vi "FipsAdjacent.vi"() -> (11 "Fips":i32[](array[numeric]))   [LabVIEW 2017] (continued)
Perce County, ID\"\t16069\n\"Idaho County, ID\"\t16049\t\"Valley County, ID\"\t16085\n\"Idaho County, ID\"\t16049\t\"Missoula County, MT\"\t30063\n\"Idaho County, ID\"\t16049\t\"Ravalli County, MT\"\t30081\n\"Idaho County, ID\"\t16049\t\"Wallowa County, OR\"\t41063\n\"Jefferson County, ID\"\t16051\t\"Bingham County, ID\"\t16011\n\"Jefferson County, ID\"\t16051\t\"Bonneville County, ID\"\t16019\n\"Jefferson County, ID\"\t16051\t\"Butte County, ID\"\t16023\n\"Jefferson County, ID\"\t16051\t\"Clark County, ID\"\t16033\n\"Jefferson County, ID\"\t16051\t\"Fremont County, ID\"\t16043\n\"Jefferson County, ID\"\t16051\t\"Jefferson County, ID\"\t16051\n\"Jefferson County, ID\"\t16051\t\"Madison County, ID\"\t16065\n\"Jerome County, ID\"\t16053\t\"Cassia County, ID\"\t16031\n\"Jerome County, ID\"\t16053\t\"Gooding County, ID\"\t16047\n\"Jerome County, ID\"\t16053\t\"Jerome County, ID\"\t16053\n\"Jerome County, ID\"\t16053\t\"Lincoln County, ID\"\t16063\n\"Jerome County, ID\"\t16053\t\"Minidoka County, ID\"\t16067\n\"Jerome County, ID\"\t16053\t\"Twin Falls County, ID\"\t16083\n\"Kootenai County, ID\"\t16055\t\"Benewah County, ID\"\t16009\n\"Kootenai County, ID\"\t16055\t\"Bonner County, ID\"\t16017\n\"Kootenai County, ID\"\t16055\t\"Kootenai County, ID\"\t16055\n\"Kootenai County, ID\"\t16055\t\"Shoshone County, ID\"\t16079\n\"Kootenai County, ID\"\t16055\t\"Spokane County, WA\"\t53063\n\"Latah County, ID\"\t16057\t\"Benewah County, ID\"\t16009\n\"Latah County, ID\"\t16057\t\"Clearwater County, ID\"\t16035\n\"Latah County, ID\"\t16057\t\"Latah County, ID\"\t16057\n\"Latah County, ID\"\t16057\t\"Nez Perce County, ID\"\t16069\n\"Latah County, ID\"\t16057\t\"Shoshone County, ID\"\t16079\n\"Latah County, ID\"\t16057\t\"Whitman County, WA\"\t53075\n\"Lemhi County, ID\"\t16059\t\"Butte County, ID\"\t16023\n\"Lemhi County, ID\"\t16059\t\"Clark County, ID\"\t16033\n\"Lemhi County, ID\"\t16059\t\"Custer County, ID\"\t16037\n\"Lemhi County, ID\"\t16059\t\"Idaho County, ID\"\t16049\n\"Lemhi County, ID\"\t16059\t\"Lemhi County, ID\"\t16059\n\"Lemhi County, ID\"\t16059\t\"Valley County, ID\"\t16085\n\"Lemhi County, ID\"\t16059\t\"Beaverhead County, MT\"\t30001\n\"Lemhi County, ID\"\t16059\t\"Ravalli County, MT\"\t30081\n\"Lewis County, ID\"\t16061\t\"Clearwater County, ID\"\t16035\n\"Lewis County, ID\"\t16061\t\"Idaho County, ID\"\t16049\n\"Lewis County, ID\"\t16061\t\"Lewis County, ID\"\t16061\n\"Lewis County, ID\"\t16061\t\"Nez Perce County, ID\"\t16069\n\"Lincoln County, ID\"\t16063\t\"Blaine County, ID\"\t16013\n\"Lincoln County, ID\"\t16063\t\"Camas County, ID\"\t16025\n\"Lincoln County, ID\"\t16063\t\"Gooding County, ID\"\t16047\n\"Lincoln County, ID\"\t16063\t\"Jerome County, ID\"\t16053\n\"Lincoln County, ID\"\t16063\t\"Lincoln County, ID\"\t16063\n\"Lincoln County, ID\"\t16063\t\"Minidoka County, ID\"\t16067\n\"Madison County, ID\"\t16065\t\"Bonneville County, ID\"\t16019\n\"Madison County, ID\"\t16065\t\"Fremont County, ID\"\t16043\n\"Madison County, ID\"\t16065\t\"Jefferson County, ID\"\t16051\n\"Madison County, ID\"\t16065\t\"Madison County, ID\"\t16065\n\"Madison County, ID\"\t16065\t\"Teton County, ID\"\t16081\n\"Minidoka County, ID\"\t16067\t\"Blaine County, ID\"\t16013\n\"Minidoka County, ID\"\t16067\t\"Cassia County, ID\"\t16031\n\"Minidoka County, ID\"\t16067\t\"Jerome County, ID\"\t16053\n\"Minidoka County, ID\"\t16067\t\"Lincoln County, ID\"\t16063\n\"Minidoka County, ID\"\t16067\t\"Minidoka County, ID\"\t16067\n\"Nez Perce County, ID\"\t16069\t\"Clearwater County, ID\"\t16035\n\"Nez Perce County, ID\"\t16069\t\"Idaho County, ID\"\t16049\n\"Nez Perce County, ID\"\t16069\t\"Latah County, ID\"\t16057\n\"Nez Perce County, ID\"\t16069\t\"Lewis County, ID\"\t16061\n\"Nez Perce County, ID\"\t16069\t\"Nez Perce County, ID\"\t16069\n\"Nez Perce County, ID\"\t16069\t\"Wallowa County, OR\"\t41063\n\"Nez Perce County, ID\"\t16069\t\"Asotin County, WA\"\t53003\n\"Nez Perce County, ID\"\t16069\t\"Whitman County, WA\"\t53075\n\"Oneida County, ID\"\t16071\t\"Bannock County, ID\"\t16005\n\"Oneida County, ID\"\t16071\t\"Cassia County, ID\"\t16031\n\"Oneida County, ID\"\t16071\t\"Franklin County, ID\"\t16041\n\"Oneida County, ID\"\t16071\t\"Oneida County, ID\"\t16071\n\"Oneida County, ID\"\t16071\t\"Power County, ID\"\t16077\n\"Oneida County, ID\"\t16071\t\"Box Elder County, UT\"\t49003\n\"Oneida County, ID\"\t16071\t\"Cache County, UT\"\t49005\n\"Owyhee County, ID\"\t16073\t\"Ada County, ID\"\t16001\n\"Owyhee County, ID\"\t16073\t\"Canyon County, ID\"\t16027\n\"Owyhee County, ID\"\t16073\t\"Elmore County, ID\"\t16039\n\"Owyhee County, ID\"\t16073\t\"Owyhee County, ID\"\t16073\n\"Owyhee County, ID\"\t16073\t\"Twin Falls County, ID\"\t16083\n\"Owyhee County, ID\"\t16073\t\"Elko County, NV\"\t32007\n\"Owyhee County, ID\"\t16073\t\"Humboldt County, NV\"\t32013\n\"Owyhee County, ID\"\t16073\t\"Malheur County, OR\"\t41045\n\"Payette County, ID\"\t16075\t\"Canyon County, ID\"\t16027\n\"Payette County, ID\"\t16075\t\"Gem County, ID\"\t16045\n\"Payette County, ID\"\t16075\t\"Payette County, ID\"\t16075\n\"Payette County, ID\"\t16075\t\"Washington County, ID\"\t16087\n\"Payette County, ID\"\t16075\t\"Malheur County, OR\"\t41045\n\"Power County, ID\"\t16077\t\"Bannock County, ID\"\t16005\n\"Power County, ID\"\t16077\t\"Bingham County, ID\"\t16011\n\"Power County, ID\"\t16077\t\"Blaine County, ID\"\t16013\n\"Power County, ID\"\t16077\t\"Cassia County, ID\"\t16031\n\"Power County, ID\"\t16077\t\"Oneida County, ID\"\t16071\n\"Power County, ID\"\t16077\t\"Power County, ID\"\t16077\n\"Shoshone County, ID\"\t16079\t\"Benewah County, ID\"\t16009\n\"Shoshone County, ID\"\t16079\t\"Bonner County, ID\"\t16017\n\"Shoshone County, ID\"\t16079\t\"Clearwater County, ID\"\t16035\n\"Shoshone County, ID\"\t16079\t\"Kootenai County, ID\"\t16055\n\"Shoshone County, ID\"\t16079\t\"Latah County, ID\"\t16057\n\"Shoshone County, ID\"\t16079\t\"Shoshone County, ID\"\t16079\n\"Shoshone County, ID\"\t16079\t\"Mineral County, MT\"\t30061\n\"Shoshone County, ID\"\t16079\t\"Sanders County, MT\"\t30089\n\"Teton County, ID\"\t16081\t\"Bonneville County, ID\"\t16019\n\"Teton County, ID\"\t16081\t\"Fremont County, ID\"\t16043\n\"Teton County, ID\"\t16081\t\"Madison County, ID\"\t16065\n\"Teton County, ID\"\t16081\t\"Teton County, ID\"\t16081\n\"Teton County, ID\"\t16081\t\"Teton County, WY\"\t56039\n\"Twin Falls County, ID\"\t16083\t\"Cassia County, ID\"\t16031\n\"Twin Falls County, ID\"\t16083\t\"Elmore County, ID\"\t16039\n\"Twin Falls County, ID\"\t16083\t\"Gooding County, ID\"\t16047\n\"Twin Falls County, ID\"\t16083\t\"Jerome County, ID\"\t16053\n\"Twin Falls County, ID\"\t16083\t\"Owyhee County, ID\"\t16073\n\"Twin Falls County, ID\"\t16083\t\"Twin Falls County, ID\"\t16083\n\"Twin Falls County, ID\"\t16083\t\"Elko County, NV\"\t32007\n\"Valley County, ID\"\t16085\t\"Adams County, ID\"\t16003\n\"Valley County, ID\"\t16085\t\"Boise County, ID\"\t16015\n\"Valley County, ID\"\t16085\t\"Custer County, ID\"\t16037\n\"Valley County, ID\"\t16085\t\"Gem County, ID\"\t16045\n\"Valley County, ID\"\t16085\t\"Idaho County, ID\"\t16049\n\"Valley County, ID\"\t16085\t\"Lemhi County, ID\"\t16059\n\"Valley County, ID\"\t16085\t\"Valley County, ID\"\t16085\n\"Washington County, ID\"\t16087\t\"Adams County, ID\"\t16003\n\"Washington County, ID\"\t16087\t\"Gem County, ID\"\t16045\n\"Washington County, ID\"\t16087\t\"Payette County, ID\"\t16075\n\"Washington County, ID\"\t16087\t\"Washington County, ID\"\t16087\n\"Washington County, ID\"\t16087\t\"Baker County, OR\"\t41001\n\"Washington County, ID\"\t16087\t\"Malheur County, OR\"\t41045\n\"Adams County, IL\"\t17001\t\"Adams County, IL\"\t17001\n\"Adams County, IL\"\t17001\t\"Brown County, IL\"\t17009\n\"Adams County, IL\"\t17001\t\"Hancock County, IL\"\t17067\n\"Adams County, IL\"\t17001\t\"Pike County, IL\"\t17149\n\"Adams County, IL\"\t17001\t\"Schuyler County, IL\"\t17169\n\"Adams County, IL\"\t17001\t\"Lewis County, MO\"\t29111\n\"Adams County, IL\"\t17001\t\"Marion County, MO\"\t29127\n\"Alexander County, IL\"\t17003\t\"Alexander County, IL\"\t17003\n\"Alexander County, IL\"\t17003\t\"Pulaski County, IL\"\t17153\n\"Alexander County, IL\"\t17003\t\"Union County, IL\"\t17181\n\"Alexander County, IL\"\t17003\t\"Ballard County, KY\"\t21007\n\"Alexander County, IL\"\t17003\t\"Cape Girardeau County, MO\"\t29031\n\"Alexander County, IL\"\t17003\t\"Mississippi County, MO\"\t29133\n\"Alexander County, IL\"\t17003\t\"Scott County, MO\"\t29201\n\"Bond County, IL\"\t17005\t\"Bond County, IL\"\t17005\n\"Bond County, IL\"\t17005\t\"Clinton County, IL\"\t17027\n\"Bond County, IL\"\t17005\t\"Fayette County, IL\"\t17051\n\"Bond County, IL\"\t17005\t\"Madison County, IL\"\t17119\n\"Bond County, IL\"\t17005\t\"Montgomery County, IL\"\t17135\n\"Boone County, IL\"\t17007\t\"Boone County, IL\"\t17007\n\"Boone County, IL\"\t17007\t\"DeKalb County, IL\"\t17037\n\"Boone County, IL\"\t17007\t\"McHenry County, IL\"\t17111\n\"Boone County, IL\"\t17007\t\"Ogle County, IL\"\t17141\n\"Boone County, IL\"\t17007\t\"Winnebago County, IL\"\t17201\n\"Boone County, IL\"\t17007\t\"Rock County, WI\"\t55105\n\"Boone County, IL\"\t17007\t\"Walworth County, WI\"\t55127\n\"Brown County, IL\"\t17009\t\"Adams County, IL\"\t17001\n\"Brown County, IL\"\t17009\t\"Brown County, IL\"\t17009\n\"Brown County, IL\"\t17009\t\"Cass County, IL\"\t17017\n\"Brown County, IL\"\t17009\t\"Morgan County, IL\"\t17137\n\"Brown County, IL\"\t17009\t\"Pike County, IL\"\t17149\n\"Brown County, IL\"\t17009\t\"Schuyler County, IL\"\t17169\n\"Bureau County, IL\"\t17011\t\"Bureau County, IL\"\t17011\n\"Bureau County, IL\"\t17011\t\"Henry County, IL\"\t17073\n\"Bureau County, IL\"\t17011\t\"LaSalle County, IL\"\t17099\n\"Bureau County, IL\"\t17011\t\"Lee County, IL\"\t17103\n\"Bureau County, IL\"\t17011\t\"Marshall County, IL\"\t17123\n\"Bureau County, IL\"\t17011\t\"Putnam County, IL\"\t17155\n\"Bureau County, IL\"\t17011\t\"Stark County, IL\"\t17175\n\"Bureau County, IL\"\t17011\t\"Whiteside County, IL\"\t17195\n\"Calhoun County, IL\"\t17013\t\"Calhoun County, IL\"\t17013\n\"Calhoun County, IL\"\t17013\t\"Greene County, IL\"\t17061\n\"Calhoun County, IL\"\t17013\t\"Jersey County, IL\"\t17083\n\"Calhoun County, IL\"\t17013\t\"Pike County, IL\"\t17149\n\"Calhoun County, IL\"\t17013\t\"Lincoln County, MO\"\t29113\n\"Calhoun County, IL\"\t17013\t\"Pike County, MO\"\t29163\n\"Calhoun County, IL\"\t17013\t\"St. Charles County, MO\"\t29183\n\"Carroll County, IL\"\t17015\t\"Carroll County, IL\"\t17015\n\"Carroll County, IL\"\t17015\t\"Jo Daviess County, IL\"\t17085\n\"Carroll County, IL\"\t17015\t\"Ogle County, IL\"\t17141\n\"Carroll County, IL\"\t17015\t\"Stephenson County, IL\"\t17177\n\"Carroll County, IL\"\t17015\t\"Whiteside County, IL\"\t17195\n\"Carroll County, IL\"\t17015\t\"Clinton County, IA\"\t19045\n\"Carroll County, IL\"\t17015\t\"Jackson County, IA\"\t19097\n\"Cass County, IL\"\t17017\t\"Brown County, IL\"\t17009\n\"Cass County, IL\"\t17017\t\"Cass County, IL\"\t17017\n\"Cass County, IL\"\t17017\t\"Mason County, IL\"\t17125\n\"Cass County, IL\"\t17017\t\"Menard County, IL\"\t17129\n\"Cass County, IL\"\t17017\t\"Morgan County, IL\"\t17137\n\"Cass County, IL\"\t17017\t\"Sangamon County, IL\"\t17167\n\"Cass County, IL\"\t17017\t\"Schuyler County, IL\"\t17169\n\"Champaign County, IL\"\t17019\t\"Champaign County, IL\"\t17019\n\"Champaign County, IL\"\t17019\t\"Douglas County, IL\"\t17041\n\"Champaign County, IL\"\t17019\t\"Edgar County, IL\"\t17045\n\"Champaign County, IL\"\t17019\t\"Ford County, IL\"\t17053\n\"Champaign County, IL\"\t17019\t\"McLean County, IL\"\t17113\n\"Champaign County, IL\"\t17019\t\"Piatt County, IL\"\t17147\n\"Champaign County, IL\"\t17019\t\"Vermilion County, IL\"\t17183\n\"Christian County, IL\"\t17021\t\"Christian County, IL\"\t17021\n\"Christian County, IL\"\t17021\t\"Macon County, IL\"\t17115\n\"Christian County, IL\"\t17021\t\"Montgomery County, IL\"\t17135\n\"Christian County, IL\"\t17021\t\"Sangamon County, IL\"\t17167\n\"Christian County, IL\"\t17021\t\"Shelby County, IL\"\t17173\n\"Clark County, IL\"\t17023\t\"Clark County, IL\"\t17023\n\"Clark County, IL\"\t17023\t\"Coles County, IL\"\t17029\n\"Clark County, IL\"\t17023\t\"Crawford County, IL\"\t17033\n\"Clark County, IL\"\t17023\t\"Cumberland County, IL\"\t17035\n\"Clark County, IL\"\t17023\t\"Edgar County, IL\"\t17045\n\"Clark County, IL\"\t17023\t\"Jasper County, IL\"\t17079\n\"Clark County, IL\"\t17023\t\"Sullivan County, IN\"\t18153\n\"Clark County, IL\"\t17023\t\"Vigo County, IN\"\t18167\n\"Clay County, IL\"\t17025\t\"Clay County, IL\"\t17025\n\"Clay County, IL\"\t17025\t\"Effingham County, IL\"\t17049\n\"Clay County, IL\"\t17025\t\"Fayette County, IL\"\t17051\n\"Clay County, IL\"\t17025\t\"Jasper County, IL\"\t17079\n\"Clay County, IL\"\t17025\t\"Marion County, IL\"\t17121\n\"Clay County, IL\"\t17025\t\"Richland County, IL\"\t17159\n\"Clay County, IL\"\t17025\t\"Wayne County, IL\"\t17191\n\"Clinton County, IL\"\t17027\t\"Bond County, IL\"\t17005\n\"Clinton County, IL\"\t17027\t\"Clinton County, IL\"\t17027\n\"Clinton County, IL\"\t17027\t\"Fayette County, IL\"\t17051\n\"Clinton County, IL\"\t17027\t\"Madison County, IL\"\t17119\n\"Clinton County, IL\"\t17027\t\"Marion County, IL\"\t17121\n\"Clinton County, IL\"\t17027\t\"St. Clair County, IL\"\t17163\n\"Clinton County, IL\"\t17027\t\"Washington County, IL\"\t17189\n\"Coles County, IL\"\t17029\t\"Clark County, IL\"\t17023\n\"Coles County, IL\"\t17029\t\"Coles County, IL\"\t17029\n\"Coles County, IL\"\t17029\t\"Cumberland County, IL\"\t17035\n\"Coles County, IL\"\t17029\t\"Douglas County, IL\"\t17041\n\"Coles County, IL\"\t17029\t\"Edgar County, IL\"\t17045\n\"Coles County, IL\"\t17029\t\"Moultrie County, IL\"\t17139\n\"Coles County, IL\"\t17029\t\"Shelby County, IL\"\t17173\n\"Cook County, IL\"\t17031\t\"Cook County, IL\"\t17031\n\"Cook County, IL\"\t17031\t\"DuPage County, IL\"\t17043\n\"Cook County, IL\"\t17031\t\"Kane County, IL\"\t17089\n\"Cook County, IL\"\t17031\t\"Lake County, IL\"\t17097\n\"Cook County, IL\"\t17031\t\"McHenry County, IL\"\t17111\n\"Cook County, IL\"\t17031\t\"Will County, IL\"\t17197\n\"Cook County, IL\"\t17031\t\"Lake County, IN\"\t18089\n\"Cook County, IL\"\t17031\t\"Porter County, IN\"\t18127\n\"Cook County, IL\"\t17031\t\"Berrien County, MI\"\t26021\n\"Crawford County, IL\"\t17033\t\"Clark County, IL\"\t17023\n\"Crawford County, IL\"\t17033\t\"Crawford County, IL\"\t17033\n\"Crawford County, IL\"\t17033\t\"Jasper County, IL\"\t17079\n\"Crawford County, IL\"\t17033\t\"Lawrence County, IL\"\t17101\n\"Crawford County, IL\"\t17033\t\"Richland County, IL\"\t17159\n\"Crawford County, IL\"\t17033\t\"Knox County, IN\"\t18083\n\"Crawford County, IL\"\t17033\t\"Sullivan County, IN\"\t18153\n\"Cumberland County, IL\"\t17035\t\"Clark County, IL\"\t17023\n\"Cumberland County, IL\"\t17035\t\"Coles County, IL\"\t17029\n\"Cumberland County, IL\"\t17035\t\"Cumberland County, IL\"\t17035\n\"Cumberland County, IL\"\t17035\t\"Effingham County, IL\"\t17049\n\"Cumberland County, IL\"\t17035\t\"Jasper County, IL\"\t17079\n\"Cumberland County, IL\"\t17035\t\"Shelby County, IL\"\t17173\n\"DeKalb County, IL\"\t17037\t\"Boone County, IL\"\t17007\n\"DeKalb County, IL\"\t17037\t\"DeKalb County, IL\"\t17037\n\"DeKalb County, IL\"\t17037\t\"Kane County, IL\"\t17089\n\"DeKalb County, IL\"\t17037\t\"Kendall County, IL\"\t17093\n\"DeKalb County, IL\"\t17037\t\"LaSalle County, IL\"\t17099\n\"DeKalb County, IL\"\t17037\t\"Lee County, IL\"\t17103\n\"DeKalb County, IL\"\t17037\t\"McHenry County, IL\"\t17111\n\"DeKalb County, IL\"\t17037\t\"Ogle County, IL\"\t17141\n\"DeKalb County, IL\"\t17037\t\"Winnebago County, IL\"\t17201\n\"De Witt County, IL\"\t17039\t\"De Witt County, IL\"\t17039\n\"De Witt County, IL\"\t17039\t\"Logan County, IL\"\t17107\n\"De Witt County, IL\"\t17039\t\"McLean County, IL\"\t17113\n\"De Witt County, IL\"\t17039\t\"Macon County, IL\"\t17115\n\"De Witt County, IL\"\t17039\t\"Piatt County, IL\"\t17147\n\"Douglas County, IL\"\t17041\t\"Champaign County, IL\"\t17019\n\"Douglas County, IL\"\t17041\t\"Coles County, IL\"\t17029\n\"Douglas County, IL\"\t17041\t\"Douglas County, IL\"\t17041\n\"Douglas County, IL\"\t17041\t\"Edgar County, IL\"\t17045\n\"Douglas County, IL\"\t17041\t\"Moultrie County, IL\"\t17139\n\"Douglas County, IL\"\t17041\t\"Piatt County, IL\"\t17147\n\"Douglas County, IL\"\t17041\t\"Vermilion County, IL\"\t17183\n\"DuPage County, IL\"\t17043\t\"Cook County, IL\"\t17031\n\"DuPage County, IL\"\t17043\t\"DuPage County, IL\"\t17043\n\"DuPage County, IL\"\t17043\t\"Kane County, IL\"\t17089\n\"DuPage County, IL\"\t17043\t\"Kendall County, IL\"\t17093\n\"DuPage County, IL\"\t17043\t\"Will County, IL\"\t17197\n\"Edgar County, IL\"\t17045\t\"Champaign County, IL\"\t17019\n\"Edgar County, IL\"\t17045\t\"Clark County, IL\"\t17023\n\"Edgar County, IL\"\t17045\t\"Coles County, IL\"\t17029\n\"Edgar County, IL\"\t17045\t\"Douglas County, IL\"\t17041\n\"Edgar County, IL\"\t17045\t\"Edgar County, IL\"\t17045\n\"Edgar County, IL\"\t17045\t\"Vermilion County, IL\"\t17183\n\"Edgar County, IL\"\t17045\t\"Vermillion County, IN\"\t18165\n\"Edgar County, IL\"\t17045\t\"Vigo County, IN\"\t18167\n\"Edwards County, IL\"\t17047\t\"Edwards County, IL\"\t17047\n\"Edwards County, IL\"\t17047\t\"Richland County, IL\"\t17159\n\"Edwards County, IL\"\t17047\t\"Wabash County, IL\"\t17185\n\"Edwards County, IL\"\t17047\t\"Wayne County, IL\"\t17191\n\"Edwards County, IL\"\t17047\t\"White County, IL\"\t17193\n\"Effingham County, IL\"\t17049\t\"Clay County, IL\"\t17025\n\"Effingham County, IL\"\t17049\t\"Cumberland County, IL\"\t17035\n\"Effingham County, IL\"\t17049\t\"Effingham County, IL\"\t17049\n\"Effingham County, IL\"\t17049\t\"Fayette County, IL\"\t17051\n\"Effingham County, IL\"\t17049\t\"Jasper County, IL\"\t17079\n\"Effingham County, IL\"\t17049\t\"Shelby County, IL\"\t17173\n\"Fayette County, IL\"\t17051\t\"Bond County, IL\"\t17005\n\"Fayette County, IL\"\t17051\t\"Clay County, IL\"\t17025\n\"Fayette County, IL\"\t17051\t\"Clinton County, IL\"\t17027\n\"Fayette County, IL\"\t17051\t\"Effingham County, IL\"\t17049\n\"Fayette County, IL\"\t17051\t\"Fayette County, IL\"\t17051\n\"Fayette County, IL\"\t17051\t\"Marion County, IL\"\t17121\n\"Fayette County, IL\"\t17051\t\"Montgomery County, IL\"\t17135\n\"Fayette County, IL\"\t17051\t\"Shelby County, IL\"\t17173\n\"Ford County, IL\"\t17053\t\"Champaign County, IL\"\t17019\n\"Ford County, IL\"\t17053\t\"Ford County, IL\"\t17053\n\"Ford County, IL\"\t17053\t\"Iroquois County, IL\"\t17075\n\"Ford County, IL\"\t17053\t\"Kankakee County, IL\"\t17091\n\"Ford County, IL\"\t17053\t\"Livingston County, IL\"\t17105\n\"Ford County, IL\"\t17053\t\"McLean County, IL\"\t17113\n\"Ford County, IL\"\t17053\t\"Vermilion County, IL\"\t17183\n\"Franklin County, IL\"\t17055\t\"Franklin County, IL\"\t17055\n\"Franklin County, IL\"\t17055\t\"Hamilton County, IL\"\t17065\n\"Franklin County, IL\"\t17055\t\"Jackson County, IL\"\t17077\n\"Franklin County, IL\"\t17055\t\"Jefferson County, IL\"\t17081\n\"Franklin County, IL\"\t17055\t\"Perry County, IL\"\t17145\n\"Franklin County, IL\"\t17055\t\"Saline County, IL\"\t17165\n\"Franklin County, IL\"\t17055\t\"Williamson County, IL\"\t17199\n\"Fulton County, IL\"\t17057\t\"Fulton County, IL\"\t17057\n\"Fulton County, IL\"\t17057\t\"Knox County, IL\"\t17095\n\"Fulton County, IL\"\t17057\t\"McDonough County, IL\"\t17109\n\"Fulton County, IL\"\t17057\t\"Mason County, IL\"\t17125\n\"Fulton County, IL\"\t17057\t\"Peoria County, IL\"\t17143\n\"Fulton County, IL\"\t17057\t\"Schuyler County, IL\"\t17169\n\"Fulton County, IL\"\t17057\t\"Tazewell County, IL\"\t17179\n\"Fulton County, IL\"\t17057\t\"Warren County, IL\"\t17187\n\"Gallatin County, IL\"\t17059\t\"Gallatin County, IL\"\t17059\n\"Gallatin County, IL\"\t17059\t\"Hamilton County, IL\"\t17065\n\"Gallatin County, IL\"\t17059\t\"Hardin County, IL\"\t17069\n\"Gallatin County, IL\"\t17059\t\"Saline County, IL\"\t17165\n\"Gallatin County, IL\"\t17059\t\"White County, IL\"\t17193\n\"Gallatin County, IL\"\t17059\t\"Posey County, IN\"\t18129\n\"Gallatin County, IL\"\t17059\t\"Union County, KY\"\t21225\n\"Greene County, IL\"\t17061\t\"Calhoun County, IL\"\t17013\n\"Greene County, IL\"\t17061\t\"Greene County, IL\"\t17061\n\"Greene County, IL\"\t17061\t\"Jersey County, IL\"\t17083\n\"Greene County, IL\"\t17061\t\"Macoupin County, IL\"\t17117\n\"Greene County, IL\"\t17061\t\"Morgan County, IL\"\t17137\n\"Greene County, IL\"\t17061\t\"Pike County, IL\"\t17149\n\"Greene County, IL\"\t17061\t\"Scott County, IL\"\t17171\n\"Grundy County, IL\"\t17063\t\"Grundy County, IL\"\t17063\n\"Grundy County, IL\"\t17063\t\"Kankakee County, IL\"\t17091\n\"Grundy County, IL\"\t17063\t\"Kendall County, IL\"\t17093\n\"Grundy County, IL\"\t17063\t\"LaSalle County, IL\"\t17099\n\"Grundy County, IL\"\t17063\t\"Livingston County, IL\"\t17105\n\"Grundy County, IL\"\t17063\t\"Will County, IL\"\t17197\n\"Hamilton County, IL\"\t17065\t\"Franklin County, IL\"\t17055\n\"Hamilton County, IL\"\t17065\t\"Gallatin County, IL\"\t17059\n\"Hamilton County, IL\"\t17065\t\"Hamilton County, IL\"\t17065\n\"Hamilton County, IL\"\t17065\t\"Jefferson County, IL\"\t17081\n\"Hamilton County, IL\"\t17065\t\"Saline County, IL\"\t17165\n\"Hamilton County, IL\"\t17065\t\"Wayne County, IL\"\t17191\n\"Hamilton County, IL\"\t17065\t\"White County, IL\"\t17193\n\"Hancock County, IL\"\t17067\t\"Adams County, IL\"\t17001\n\"Hancock County, IL\"\t17067\t\"Hancock County, IL\"\t17067\n\"Hancock County, IL\"\t17067\t\"Henderson County, IL\"\t17071\n\"Hancock County, IL\"\t17067\t\"McDonough County, IL\"\t17109\n\"Hancock County, IL\"\t17067\t\"Schuyler County, IL\"\t17169\n\"Hancock County, IL\"\t17067\t\"Lee County, IA\"\t19111\n\"Hancock County, IL\"\t17067\t\"Clark County, MO\"\t29045\n\"Hancock County, IL\"\t17067\t\"Lewis County, MO\"\t29111\n\"Hardin County, IL\"\t17069\t\"Gallatin County, IL\"\t17059\n\"Hardin County, IL\"\t17069\t\"Hardin County, IL\"\t17069\n\"Hardin County, IL\"\t17069\t\"Pope County, IL\"\t17151\n\"Hardin County, IL\"\t17069\t\"Saline County, IL\"\t17165\n\"Hardin County, IL\"\t17069\t\"Crittenden County, KY\"\t21055\n\"Hardin County, IL\"\t17069\t\"Livingston County, KY\"\t21139\n\"Hardin County, IL\"\t17069\t\"Union County, KY\"\t21225\n\"Henderson County, IL\"\t17071\t\"Hancock County, IL\"\t17067\n\"Henderson County, IL\"\t17071\t\"Henderson County, IL\"\t17071\n\"Henderson County, IL\"\t17071\t\"McDonough County, IL\"\t17109\n\"Henderson County, IL\"\t17071\t\"Mercer County, IL\"\t17131\n\"Henderson County, IL\"\t17071\t\"Warren County, IL\"\t17187\n\"Henderson County, IL\"\t17071\t\"Des Moines County, IA\"\t19057\n\"Henderson County, IL\"\t17071\t\"Lee County, IA\"\t19111\n\"Henry County, IL\"\t17073\t\"Bureau County, IL\"\t17011\n\"Henry County, IL\"\t17073\t\"Henry County, IL\"\t17073\n\"Henry County, IL\"\t17073\t\"Knox County, IL\"\t17095\n\"Henry County, IL\"\t17073\t\"Mercer County, IL\"\t17131\n\"Henry County, IL\"\t17073\t\"Rock Island County, IL\"\t17161\n\"Henry County, IL\"\t17073\t\"Stark County, IL\"\t17175\n\"Henry County, IL\"\t17073\t\"Whiteside County, IL\"\t17195\n\"Iroquois County, IL\"\t17075\t\"Ford County, IL\"\t17053\n\"Iroquois County, IL\"\t17075\t\"Iroquois County, IL\"\t17075\n\"Iroquois County, IL\"\t17075\t\"Kankakee County, IL\"\t17091\n\"Iroquois County, IL\"\t17075\t\"Vermilion County, IL\"\t17183\n\"Iroquois County, IL\"\t17075\t\"Benton County, IN\"\t18007\n\"Iroquois County, IL\"\t17075\t\"Newton County, IN\"\t18111\n\"Jackson County, IL\"\t17077\t\"Franklin County, IL\"\t17055\n\"Jackson County, IL\"\t17077\t\"Jackson County, IL\"\t17077\n\"Jackson County, IL\"\t17077\t\"Perry County, IL\"\t17145\n\"Jackson County, IL\"\t17077\t\"Randolph County, IL\"\t17157\n\"Jackson County, IL\"\t17077\t\"Union County, IL\"\t17181\n\"Jackson County, IL\"\t17077\t\"Williamson County, IL\"\t17199\n\"Jackson County, IL\"\t17077\t\"Perry County, MO\"\t29157\n\"Jasper County, IL\"\t17079\t\"Clark County, IL\"\t17023\n\"Jasper County, IL\"\t17079\t\"Clay County, IL\"\t17025\n\"Jasper County, IL\"\t17079\t\"Crawford County, IL\"\t17033\n\"Jasper County, IL\"\t17079\t\"Cumberland County, IL\"\t17035\n\"Jasper County, IL\"\t17079\t\"Effingham County, IL\"\t17049\n\"Jasper County, IL\"\t17079\t\"Jasper County, IL\"\t17079\n\"Jasper County, IL\"\t17079\t\"Richland County, IL\"\t17159\n\"Jefferson County, IL\"\t17081\t\"Franklin County, IL\"\t17055\n\"Jefferson County, IL\"\t17081\t\"Hamilton County, IL\"\t17065\n\"Jefferson County, IL\"\t17081\t\"Jefferson County, IL\"\t17081\n\"Jefferson County, IL\"\t17081\t\"Marion County, IL\"\t17121\n\"Jefferson County, IL\"\t17081\t\"Perry County, IL\"\t17145\n\"Jefferson County, IL\"\t17081\t\"Washington County, IL\"\t17189\n\"Jefferson County, IL\"\t17081\t\"Wayne County, IL\"\t17191\n\"Jersey County, IL\"\t17083\t\"Calhoun County, IL\"\t17013\n\"Jersey County, IL\"\t17083\t\"Greene County, IL\"\t17061\n\"Jersey County, IL\"\t17083\t\"Jersey County, IL\"\t17083\n\"Jersey County, IL\"\t17083\t\"Macoupin County, IL\"\t17117\n\"Jersey County, IL\"\t17083\t\"Madison County, IL\"\t17119\n\"Jersey County, IL\"\t17083\t\"St. Charles County, MO\"\t29183\n\"Jo Daviess County, IL\"\t17085\t\"Carroll County, IL\"\t17015\n\"Jo Daviess County, IL\"\t17085\t\"Jo Daviess County, IL\"\t17085\n\"Jo Daviess County, IL\"\t17085\t\"Stephenson County, IL\"\t17177\n\"Jo Daviess County, IL\"\t17085\t\"Dubuque County, IA\"\t19061\n\"Jo Daviess County, IL\"\t17085\t\"Jackson County, IA\"\t19097\n\"Jo Daviess County, IL\"\t17085\t\"Grant County, WI\"\t55043\n\"Jo Daviess County, IL\"\t17085\t\"Lafayette County, WI\"\t55065\n\"Johnson County, IL\"\t17087\t\"Johnson County, IL\"\t17087\n\"Johnson County, IL\"\t17087\t\"Massac County, IL\"\t17127\n\"Johnson County, IL\"\t17087\t\"Pope County, IL\"\t17151\n\"Johnson County, IL\"\t17087\t\"Pulaski County, IL\"\t17153\n\"Johnson County, IL\"\t17087\t\"Saline County, IL\"\t17165\n\"Johnson County, IL\"\t17087\t\"Union County, IL\"\t17181\n\"Johnson County, IL\"\t17087\t\"Williamson County, IL\"\t17199\n\"Kane County, IL\"\t17089\t\"Cook County, IL\"\t17031\n\"Kane County, IL\"\t17089\t\"DeKalb County, IL\"\t17037\n\"Kane County, IL\"\t17089\t\"DuPage County, IL\"\t17043\n\"Kane County, IL\"\t17089\t\"Kane County, IL\"\t17089\n\"Kane County, IL\"\t17089\t\"Kendall County, IL\"\t17093\n\"Kane County, IL\"\t17089\t\"McHenry County, IL\"\t17111\n\"Kankakee County, IL\"\t17091\t\"Ford County, IL\"\t17053\n\"Kankakee County, IL\"\t17091\t\"Grundy County, IL\"\t17063\n\"Kankakee County, IL\"\t17091\t\"Iroquois County, IL\"\t17075\n\"Kankakee County, IL\"\t17091\t\"Kankakee County, IL\"\t17091\n\"Kankakee County, IL\"\t17091\t\"Livingston County, IL\"\t17105\n\"Kankakee County, IL\"\t17091\t\"Will County, IL\"\t17197\n\"Kankakee County, IL\"\t17091\t\"Lake County, IN\"\t18089\n\"Kankakee County, IL\"\t17091\t\"Newton County, IN\"\t18111\n\"Kendall County, IL\"\t17093\t\"DeKalb County, IL\"\t17037\n\"Kendall County, IL\"\t17093\t\"DuPage County, IL\"\t17043\n\"Kendall County, IL\"\t17093\t\"Grundy County, IL\"\t17063\n\"Kendall County, IL\"\t17093\t\"Kane County, IL\"\t17089\n\"Kendall County, IL\"\t17093\t\"Kendall County, IL\"\t17093\n\"Kendall County, IL\"\t17093\t\"LaSalle County, IL\"\t17099\n\"Kendall County, IL\"\t17093\t\"Will County, IL\"\t17197\n\"Knox County, IL\"\t17095\t\"Fulton County, IL\"\t17057\n\"Knox County, IL\"\t17095\t\"Henry County, IL\"\t17073\n\"Knox County, IL\"\t17095\t\"Knox County, IL\"\t17095\n\"Knox County, IL\"\t17095\t\"Mercer County, IL\"\t17131\n\"Knox County, IL\"\t17095\t\"Peoria County, IL\"\t17143\n\"Knox County, IL\"\t17095\t\"Stark County, IL\"\t17175\n\"Knox County, IL\"\t17095\t\"Warren County, IL\"\t17187\n\"Lake County, IL\"\t17097\t\"Cook County, IL\"\t17031\n\"Lake County, IL\"\t17097\t\"Lake County, IL\"\t17097\n\"Lake County, IL\"\t17097\t\"McHenry County, IL\"\t17111\n\"Lake County, IL\"\t17097\t\"Allegan County, MI\"\t26005\n\"Lake County, IL\"\t17097\t\"Berrien County, MI\"\t26021\n\"Lake County, IL\"\t17097\t\"Van Buren County, MI\"\t26159\n\"Lake County, IL\"\t17097\t\"Kenosha County, WI\"\t55059\n\"LaSalle County, IL\"\t17099\t\"Bureau County, IL\"\t17011\n\"LaSalle County, IL\"\t17099\t\"DeKalb County, IL\"\t17037\n\"LaSalle County, IL\"\t17099\t\"Grundy County, IL\"\t17063\n\"LaSalle County, IL\"\t17099\t\"Kendall County, IL\"\t17093\n\"LaSalle County, IL\"\t17099\t\"LaSalle County, IL\"\t17099\n\"LaSalle County, IL\"\t17099\t\"Lee County, IL\"\t17103\n\"LaSalle County, IL\"\t17099\t\"Livingston County, IL\"\t17105\n\"LaSalle County, IL\"\t17099\t\"Marshall County, IL\"\t17123\n\"LaSalle County, IL\"\t17099\t\"Putnam County, IL\"\t17155\n\"LaSalle County, IL\"\t17099\t\"Woodford County, IL\"\t17203\n\"Lawrence County, IL\"\t17101\t\"Crawford County, IL\"\t17033\n\"Lawrence County, IL\"\t17101\t\"Lawrence County, IL\"\t17101\n\"Lawrence County, IL\"\t17101\t\"Richland County, IL\"\t17159\n\"Lawrence County, IL\"\t17101\t\"Wabash County, IL\"\t17185\n\"Lawrence County, IL\"\t17101\t\"Knox County, IN\"\t18083\n\"Lee County, IL\"\t17103\t\"Bureau County, IL\"\t17011\n\"Lee County, IL\"\t17103\t\"DeKalb County, IL\"\t17037\n\"Lee County, IL\"\t17103\t\"LaSalle County, IL\"\t17099\n\"Lee County, IL\"\t17103\t\"Lee County, IL\"\t17103\n\"Lee County, IL\"\t17103\t\"Ogle County, IL\"\t17141\n\"Lee County, IL\"\t17103\t\"Whiteside County, IL\"\t17195\n\"Livingston County, IL\"\t17105\t\"Ford County, IL\"\t17053\n\"Livingston County, IL\"\t17105\t\"Grundy County, IL\"\t17063\n\"Livingston County, IL\"\t17105\t\"Kankakee County, IL\"\t17091\n\"Livingston County, IL\"\t17105\t\"LaSalle County, IL\"\t17099\n\"Livingston County, IL\"\t17105\t\"Livingston County, IL\"\t17105\n\"Livingston County, IL\"\t17105\t\"McLean County, IL\"\t17113\n\"Livingston County, IL\"\t17105\t\"Woodford County, IL\"\t17203\n\"Logan County, IL\"\t17107\t\"De Witt County, IL\"\t17039\n\"Logan County, IL\"\t17107\t\"Logan County, IL\"\t17107\n\"Logan County, IL\"\t17107\t\"McLean County, IL\"\t17113\n\"Logan County, IL\"\t17107\t\"Macon County, IL\"\t17115\n\"Logan County, IL\"\t17107\t\"Mason County, IL\"\t17125\n\"Logan County, IL\"\t17107\t\"Menard County, IL\"\t17129\n\"Logan County, IL\"\t17107\t\"Sangamon County, IL\"\t17167\n\"Logan County, IL\"\t17107\t\"Tazewell County, IL\"\t17179\n\"McDonough County, IL\"\t17109\t\"Fulton County, IL\"\t17057\n\"McDonough County, IL\"\t17109\t\"Hancock County, IL\"\t17067\n\"McDonough County, IL\"\t17109\t\"Henderson County, IL\"\t17071\n\"McDonough County, IL\"\t17109\t\"McDonough County, IL\"\t17109\n\"McDonough County, IL\"\t17109\t\"Schuyler County, IL\"\t17169\n\"McDonough County, IL\"\t17109\t\"Warren County, IL\"\t17187\n\"McHenry County, IL\"\t17111\t\"Boone County, IL\"\t17007\n\"McHenry County, IL\"\t17111\t\"Cook County, IL\"\t17031\n\"McHenry County, IL\"\t17111\t\"DeKalb County, IL\"\t17037\n\"McHenry County, IL\"\t17111\t\"Kane County, IL\"\t17089\n\"McHenry County, IL\"\t17111\t\"Lake County, IL\"\t17097\n\"McHenry County, IL\"\t17111\t\"McHenry County, IL\"\t17111\n\"McHenry County, IL\"\t17111\t\"Kenosha County, WI\"\t55059\n\"McHenry County, IL\"\t17111\t\"Walworth County, WI\"\t55127\n\"McLean County, IL\"\t17113\t\"Champaign County, IL\"\t17019\n\"McLean County, IL\"\t17113\t\"De Witt County, IL\"\t17039\n\"McLean County, IL\"\t17113\t\"Ford County, IL\"\t17053\n\"McLean County, IL\"\t17113\t\"Livingston County, IL\"\t17105\n\"McLean County, IL\"\t17113\t\"Logan County, IL\"\t17107\n\"McLean County, IL\"\t17113\t\"McLean County, IL\"\t17113\n\"McLean County, IL\"\t17113\t\"Piatt County, IL\"\t17147\n\"McLean County, IL\"\t17113\t\"Tazewell County, IL\"\t17179\n\"McLean County, IL\"\t17113\t\"Woodford County, IL\"\t17203\n\"Macon County, IL\"\t17115\t\"Christian County, IL\"\t17021\n\"Macon County, IL\"\t17115\t\"De Witt County, IL\"\t17039\n\"Macon County, IL\"\t17115\t\"Logan County, IL\"\t17107\n\"Macon County, IL\"\t17115\t\"Macon County, IL\"\t17115\n\"Macon County, IL\"\t17115\t\"Moultrie County, IL\"\t17139\n\"Macon County, IL\"\t17115\t\"Piatt County, IL\"\t17147\n\"Macon County, IL\"\t17115\t\"Sangamon County, IL\"\t17167\n\"Macon County, IL\"\t17115\t\"Shelby County, IL\"\t17173\n\"Macoupin County, IL\"\t17117\t\"Greene County, IL\"\t17061\n\"Macoupin County, IL\"\t17117\t\"Jersey County, IL\"\t17083\n\"Macoupin County, IL\"\t17117\t\"Macoupin County, IL\"\t17117\n\"Macoupin County, IL\"\t17117\t\"Madison County, IL\"\t17119\n\"Macoupin County, IL\"\t17117\t\"Montgomery County, IL\"\t17135\n\"Macoupin County, IL\"\t17117\t\"Morgan County, IL\"\t17137\n\"Macoupin County, IL\"\t17117\t\"Sangamon County, IL\"\t17167\n\"Madison County, IL\"\t17119\t\"Bond County, IL\"\t17005\n\"Madison County, IL\"\t17119\t\"Clinton County, IL\"\t17027\n\"Madison County, IL\"\t17119\t\"Jersey County, IL\"\t17083\n\"Madison County, IL\"\t17119\t\"Macoupin County, IL\"\t17117\n\"Madison County, IL\"\t17119\t\"Madison County, IL\"\t17119\n\"Madison County, IL\"\t17119\t\"Montgomery County, IL\"\t17135\n\"Madison County, IL\"\t17119\t\"St. Clair County, IL\"\t17163\n\"Madison County, IL\"\t17119\t\"St. Charles County, MO\"\t29183\n\"Madison County, IL\"\t17119\t\"St. Louis County, MO\"\t29189\n\"Madison County, IL\"\t17119\t\"St. Louis city, MO\"\t29510\n\"Marion County, IL\"\t17121\t\"Clay County, IL\"\t17025\n\"Marion County, IL\"\t17121\t\"Clinton County, IL\"\t17027\n\"Marion County, IL\"\t17121\t\"Fayette County, IL\"\t17051\n\"Marion County, IL\"\t17121\t\"Jefferson County, IL\"\t17081\n\"Marion County, IL\"\t17121\t\"Marion County, IL\"\t17121\n\"Marion County, IL\"\t17121\t\"Washington County, IL\"\t17189\n\"Marion County, IL\"\t17121\t\"Wayne County, IL\"\t17191\n\"Marshall County, IL\"\t17123\t\"Bureau County, IL\"\t17011\n\"Marshall County, IL\"\t17123\t\"LaSalle County, IL\"\t17099\n\"Marshall County, IL\"\t17123\t\"Marshall County, IL\"\t17123\n\"Marshall County, IL\"\t17123\t\"Peoria County, IL\"\t17143\n\"Marshall County, IL\"\t17123\t\"Putnam County, IL\"\t17155\n\"Marshall County, IL\"\t17123\t\"Stark County, IL\"\t17175\n\"Marshall County, IL\"\t17123\t\"Woodford County, IL\"\t17203\n\"Mason County, IL\"\t17125\t\"Cass County, IL\"\t17017\n\"Mason County, IL\"\t17125\t\"Fulton County, IL\"\t17057\n\"Mason County, IL\"\t17125\t\"Logan County, IL\"\t17107\n\"Mason County, IL\"\t17125\t\"Mason County, IL\"\t17125\n\"Mason County, IL\"\t17125\t\"Menard County, IL\"\t17129\n\"Mason County, IL\"\t17125\t\"Schuyler County, IL\"\t17169\n\"Mason County, IL\"\t17125\t\"Tazewell County, IL\"\t17179\n\"Massac County, IL\"\t17127\t\"Johnson County, IL\"\t17087\n\"Massac County, IL\"\t17127\t\"Massac County, IL\"\t17127\n\"Massac County, IL\"\t17127\t\"Pope County, IL\"\t17151\n\"Massac County, IL\"\t17127\t\"Pulaski County, IL\"\t17153\n\"Massac County, IL\"\t17127\t\"Livingston County, KY\"\t21139\n\"Massac County, IL\"\t17127\t\"McCracken County, KY\"\t21145\n\"Menard County, IL\"\t17129\t\"Cass County, IL\"\t17017\n\"Menard County, IL\"\t17129\t\"Logan County, IL\"\t17107\n\"Menard County, IL\"\t17129\t\"Mason County, IL\"\t17125\n\"Menard County, IL\"\t17129\t\"Menard County, IL\"\t17129\n\"Menard County, IL\"\t17129\t\"Sangamon County, IL\"\t17167\n\"Mercer County, IL\"\t17131\t\"Henderson County, IL\"\t17071\n\"Mercer County, IL\"\t17131\t\"Henry County, IL\"\t17073\n\"Mercer County, IL\"\t17131\t\"Knox County, IL\"\t17095\n\"Mercer County, IL\"\t17131\t\"Mercer County, IL\"\t17131\n\"Mercer County, IL\"\t17131\t\"Rock Island County, IL\"\t17161\n\"Mercer County, IL\"\t17131\t\"Warren County, IL\"\t17187\n\"Mercer County, IL\"\t17131\t\"Des Moines County, IA\"\t19057\n\"Mercer County, IL\"\t17131\t\"Louisa County, IA\"\t19115\n\"Monroe County, IL\"\t17133\t\"Monroe County, IL\"\t17133\n\"Monroe County, IL\"\t17133\t\"Randolph County, IL\"\t17157\n\"Monroe County, IL\"\t17133\t\"St. Clair County, IL\"\t17163\n\"Monroe County, IL\"\t17133\t\"Jefferson County, MO\"\t29099\n\"Monroe County, IL\"\t17133\t\"Ste. Genevieve County, MO\"\t29186\n\"Monroe County, IL\"\t17133\t\"St. Louis County, MO\"\t29189\n\"Montgomery County, IL\"\t17135\t\"Bond County, IL\"\t17005\n\"Montgomery County, IL\"\t17135\t\"Christian County, IL\"\t17021\n\"Montgomery County, IL\"\t17135\t\"Fayette County, IL\"\t17051\n\"Montgomery County, IL\"\t17135\t\"Macoupin County, IL\"\t17117\n\"Montgomery County, IL\"\t17135\t\"Madison County, IL\"\t17119\n\"Montgomery County, IL\"\t17135\t\"Montgomery County, IL\"\t17135\n\"Montgomery County, IL\"\t17135\t\"Sangamon County, IL\"\t17167\n\"Montgomery County, IL\"\t17135\t\"Shelby County, IL\"\t17173\n\"Morgan County, IL\"\t17137\t\"Brown County, IL\"\t17009\n\"Morgan County, IL\"\t17137\t\"Cass County, IL\"\t17017\n\"Morgan County, IL\"\t17137\t\"Greene County, IL\"\t17061\n\"Morgan County, IL\"\t17137\t\"Macoupin County, IL\"\t17117\n\"Morgan County, IL\"\t17137\t\"Morgan County, IL\"\t17137\n\"Morgan County, IL\"\t17137\t\"Pike County, IL\"\t17149\n\"Morgan County, IL\"\t17137\t\"Sangamon County, IL\"\t17167\n\"Morgan County, IL\"\t17137\t\"Scott County, IL\"\t17171\n\"Moultrie County, IL\"\t17139\t\"Coles County, IL\"\t17029\n\"Moultrie County, IL\"\t17139\t\"Douglas County, IL\"\t17041\n\"Moultrie County, IL\"\t17139\t\"Macon County, IL\"\t17115\n\"Moultrie County, IL\"\t17139\t\"Moultrie County, IL\"\t17139\n\"Moultrie County, IL\"\t17139\t\"Piatt County, IL\"\t17147\n\"Moultrie County, IL\"\t17139\t\"Shelby County, IL\"\t17173\n\"Ogle County, IL\"\t17141\t\"Boone County, IL\"\t17007\n\"Ogle County, IL\"\t17141\t\"Carroll County, IL\"\t17015\n\"Ogle County, IL\"\t17141\t\"DeKalb County, IL\"\t17037\n\"Ogle County, IL\"\t17141\t\"Lee County, IL\"\t17103\n\"Ogle County, IL\"\t17141\t\"Ogle County, IL\"\t17141\n\"Ogle County, IL\"\t17141\t\"Stephenson County, IL\"\t17177\n\"Ogle County, IL\"\t17141\t\"Whiteside County, IL\"\t17195\n\"Ogle County, IL\"\t17141\t\"Winnebago County, IL\"\t17201\n\"Peoria County, IL\"\t17143\t\"Fulton County, IL\"\t17057\n\"Peoria County, IL\"\t17143\t\"Knox County, IL\"\t17095\n\"Peoria County, IL\"\t17143\t\"Marshall County, IL\"\t17123\n\"Peoria County, IL\"\t17143\t\"Peoria County, IL\"\t17143\n\"Peoria County, IL\"\t17143\t\"Stark County, IL\"\t17175\n\"Peoria County, IL\"\t17143\t\"Tazewell County, IL\"\t17179\n\"Peoria County, IL\"\t17143\t\"Woodford County, IL\"\t17203\n\"Perry County, IL\"\t17145\t\"Franklin County, IL\"\t17055\n\"Perry County, IL\"\t17145\t\"Jackson County, IL\"\t17077\n\"Perry County, IL\"\t17145\t\"Jefferson County, IL\"\t17081\n\"Perry County, IL\"\t17145\t\"Perry County, IL\"\t17145\n\"Perry County, IL\"\t17145\t\"Randolph County, IL\"\t17157\n\"Perry County, IL\"\t17145\t\"Washington County, IL\"\t17189\n\"Piatt County, IL\"\t17147\t\"Champaign County, IL\"\t17019\n\"Piatt County, IL\"\t17147\t\"De Witt County, IL\"\t17039\n\"Piatt County, IL\"\t17147\t\"Douglas County, IL\"\t17041\n\"Piatt County, IL\"\t17147\t\"McLean County, IL\"\t17113\n\"Piatt County, IL\"\t17147\t\"Macon County, IL\"\t17115\n\"Piatt County, IL\"\t17147\t\"Moultrie County, IL\"\t17139\n\"Piatt County, IL\"\t17147\t\"Piatt County, IL\"\t17147\n\"Pike County, IL\"\t17149\t\"Adams County, IL\"\t17001\n\"Pike County, IL\"\t17149\t\"Brown County, IL\"\t17009\n\"Pike County, IL\"\t17149\t\"Calhoun County, IL\"\t17013\n\"Pike County, IL\"\t17149\t\"Greene County, IL\"\t17061\n\"Pike County, IL\"\t17149\t\"Morgan County, IL\"\t17137\n\"Pike County, IL\"\t17149\t\"Pike County, IL\"\t17149\n\"Pike County, IL\"\t17149\t\"Scott County, IL\"\t17171\n\"Pike County, IL\"\t17149\t\"Marion County, MO\"\t29127\n\"Pike County, IL\"\t17149\t\"Pike County, MO\"\t29163\n\"Pike County, IL\"\t17149\t\"Ralls County, MO\"\t29173\n\"Pope County, IL\"\t17151\t\"Hardin County, IL\"\t17069\n\"Pope County, IL\"\t17151\t\"Johnson County, IL\"\t17087\n\"Pope County, IL\"\t17151\t\"Massac County, IL\"\t17127\n\"Pope County, IL\"\t17151\t\"Pope County, 
